vi "Engine In - Sensor - Pedal.vi"(10 "Loop Freq (Hz)":sgl, 11 "Pedal [V]":sgl) -> (3 "Pedal [%]":sgl)   [LabVIEW 2015, in "ECS-RT.lvlib"]
uses:
  ECS-RT.lvlib
  <vilib>/ptbypt/NI_PtbyPt.lvlib
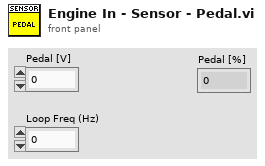
[diagram p1: front panel]
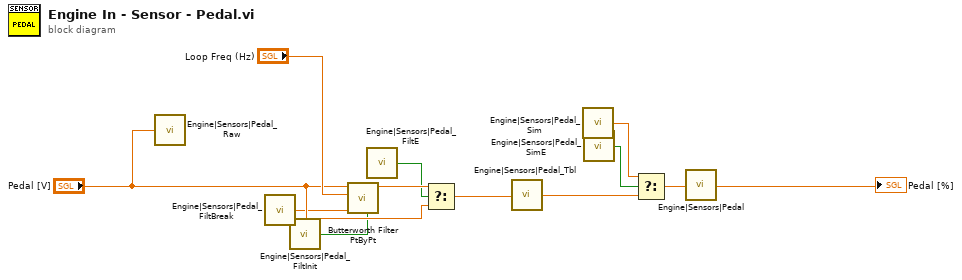
[diagram p0: block diagram]
diagram:
  n1 = call "Engine|Sensors|Pedal_Raw"("Value"="Pedal [V]") -> ()
  n2 = call "Engine|Sensors|Pedal_FiltBreak"() -> ("Value"=w4:sgl)
  n3 = call "Engine|Sensors|Pedal_FiltInit"() -> ("Value"=w7:bool)
  n4 = call <vilib>:"Butterworth Filter PtByPt.vi"("initialize"=w7, "low cutoff freq: fl"=w4, "sampling freq: fs"="Loop Freq (Hz)", "x"="Pedal [V]") -> ("Filtered x"=w6:dbl)  [unwired: 5 in, 1 out]
  n5 = call "Engine|Sensors|Pedal_FiltE"() -> ("Value"=w3:bool)
  n6 = Select(t=w6, s=w3, f="Pedal [V]") -> (s? t:f=w5:dbl)
  n7 = call "Engine|Sensors|Pedal_Tbl"("X Index"=w5) -> ("Y"=w2:sgl)
  n8 = call "Engine|Sensors|Pedal_Sim"() -> ("Value"=w8:sgl)
  n9 = call "Engine|Sensors|Pedal_SimE"() -> ("Value"=w1:bool)
  n10 = Select(t=w8, s=w1, f=w2) -> (s? t:f=w10:sgl)
  "Pedal [%]" <- w10
  n11 = call "Engine|Sensors|Pedal"("Value"=w10) -> ()
